vi "channels_to_stream.set.vi"(8 "error in (no error)":errorcluster, 10 "Channels to Stream":string[](array[string]), 11 "Nominal IO Client in":T1 format="%.0x") -> (0 "error out":errorcluster, 3 "Nominal IO Client out":T1 format="%.0x", 4 "Replaced":bool)   [LabVIEW 2024, in "Nominal Client Scripting.lvlib"]
uses:
  Nominal Client Scripting.lvlib
  <vilib>/NI VeriStand/Custom Device API/Custom Device Item Ref.ctl
  <vilib>/NI VeriStand/Custom Device API/Set Item Property (String Array).vi
  <vilib>/NI VeriStand/Custom Device API/Custom Device API.lvlib
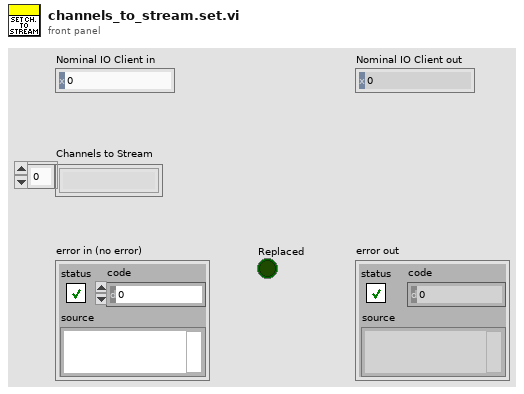
[diagram p1: front panel]
types:
  T1 = typedef "Custom Device API.lvlib/Custom Device Item Ref.ctl" = u64
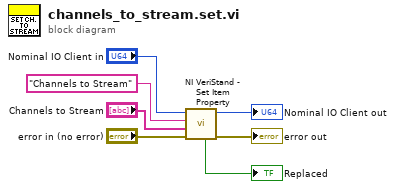
[diagram p0: block diagram]
diagram:
  n1 = call-poly <vilib>:"NI VeriStand - Set Item Property.vi"("error in (no error)"="error in (no error)", "Value"="Channels to Stream", "Property Name"="Channels to Stream", "Item Ref in"="Nominal IO Client in") -> ("error out"=→"error out":errorcluster, "Item Ref out"=→"Nominal IO Client out":T1, "Replaced"=→"Replaced":bool)  [unwired: 5 in]
